vi "missionLocation.vi"(8 "error in (no error)":errorcluster, 11 "StationKeeping in":refnum<class "StationKeeping.lvclass">) -> (0 "error out":errorcluster, 2 "element":T1 {"North" format="%#_10f"; "East" format="%#_8f"}, 3 "StationKeeping out":refnum<class "StationKeeping.lvclass">)   [LabVIEW 2013, in "StationKeeping.lvclass"]
uses:
  StationKeeping.lvclass
  Data/TypeDefs/UTM Location.ctl
  StationKeeping.lvclass/StationKeeping.ctl
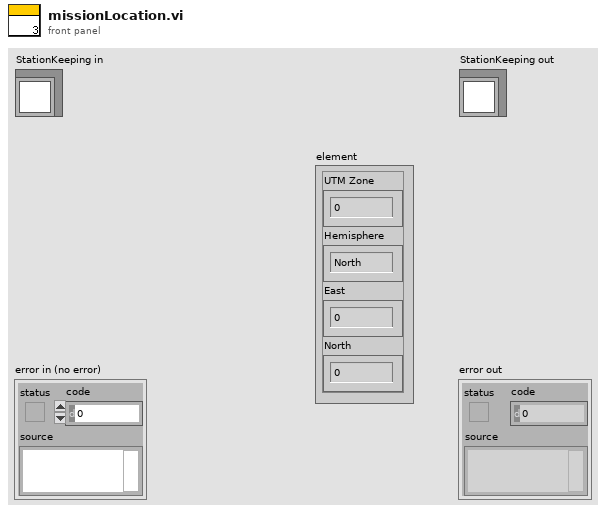
[diagram p1: front panel]
types:
  T1 = typedef "UTM Location.ctl" = cluster{"UTM Zone":dbl, "Hemisphere":enum16{"North", "South"}, "East":dbl, "North":dbl}
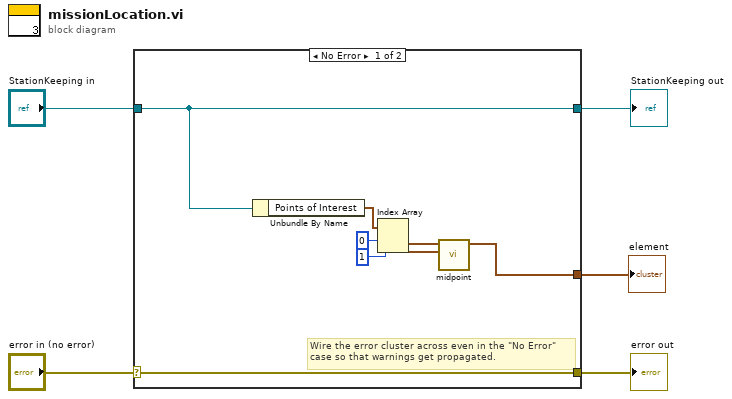
[diagram p0: block diagram]
diagram:
  n1 = case shown="No Error" "error in (no error)" {
    selector: "error in (no error)" -> [w13 w15]
    tunnel: [w13 w15] -> w4
    tunnel: [w11 w14] -> w2
    tunnel: "StationKeeping in" -> [w11 w14]
    tunnel: [w8 _] -> w1
    frame No Error {
      # "Wire the error cluster across even in the \"No Error\"\ncase so that warnings get propagated."
      n2 = Unbundle By Name(w11) -> ("Points of Interest"=w10:T1[])
      n3 = Index Array(array=w10, index #1=0 ("index"), index #2=1 ("index")) -> (element #1=w7:T1, element #2=w6:T1)
      n4 = call "midpoint.vi"("UTM Location 2"=w6, "UTM Location"=w7) -> ("UTM Location 3"=w8:T1)  [unwired: 8 in, 1 out]
    }
    frame Error {
    }
  }
  "error out" <- w4
  "StationKeeping out" <- w2
  "element" <- w1
